vi "Img_CaptureAndSaveImg.vi"(4 "error in":errorcluster, 5 "Sequence No":i32, 6 "SaveImg":bool, 7 "Image In":T1, 8 "Session In":T2) -> (0 "error out":errorcluster, 1 "Buffer Number Out":u32, 2 "Image Out":T1, 3 "Session Out":T2)   [LabVIEW 2009]
uses:
  <vilib>/userDefined/High Color/IMAQdx.ctl
  <vilib>/vision/Image Controls.llb/IMAQ Image.ctl
  <vilib>/vision/driver/NI_Vision_Acquisition_Software.lvlib
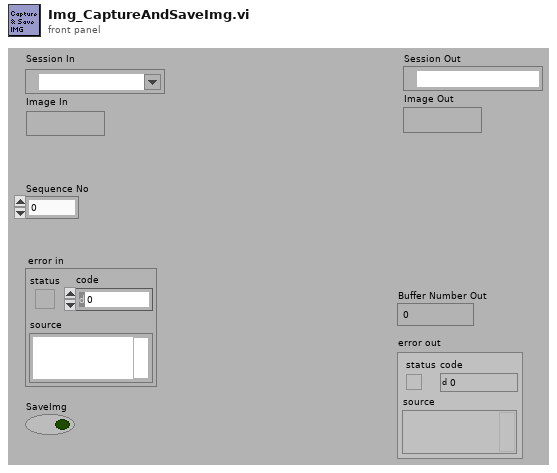
[diagram p1: front panel]
types:
  T1 = typedef "IMAQ Image.ctl" = refnum<image>
  T2 = typedef "IMAQdx.ctl" = refnum<k21>
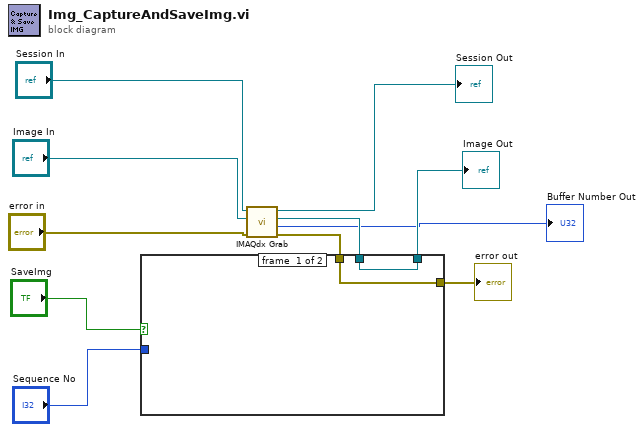
[diagram p0: block diagram]
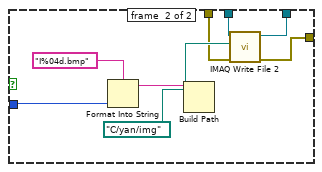
[diagram p2: hidden frame]
diagram:
  n1 = call <vilib>:"IMAQdx Grab.vi"("error in"="error in", "Image In"="Image In", "Session In"="Session In") -> ("error out"=w8:errorcluster, "Buffer Number Out"=→"Buffer Number Out":u32, "Image Out"=w4:T1, "Session Out"=→"Session Out":T2)  [unwired: 5 in]
  n2 = case shown="True" "SaveImg" {
    tunnel: w8 -> [w12 w18]
    tunnel: [w12 w17] -> w6
    tunnel: "Sequence No" -> [_ w16]
    tunnel: w4 -> [w13 w15]
    tunnel: [w13 w14] -> w2
    frame #0 {
    }
    frame #1 {
      n3 = Format Into String(format string="I%04d.bmp", w16) -> (resulting string=w21:string)  [unwired: 2 in, 1 out]
      n4 = Build Path(base path=path "C:/yan/img" ("File Path"), name or relative path=w21) -> (appended path=w19:path)
      n5 = call-poly "IMAQ Write File 2"("error in (no error)"=w18, "File Path"=w19, "Image"=w15) -> ("error out"=w17:errorcluster, "Image Out (duplicate)"=w14:T1)  [unwired: 7 in]
    }
  }
  "Image Out" <- w2
  "error out" <- w6
